vi "DAQ_E_mIO_DIO.reset.vi"(0 "i ref in":refnum<vi>, 3 "ms timeout (10000)":i32=10000, 5 "error in (no error)":errorcluster) -> (14 "i ref out":refnum<vi>, 17 "timed out":bool, 19 "error out":errorcluster)   [LabVIEW 2014, in "DAQ_E_mIO_DIO.lvlib"]
doc: "Sets all bits of the digital output port to 0.\n\nLicense Agreement for this software:\n\nCopyright (C)\nGesellschaft für Schwerionenforschung, GSI\nPlanckstr. 1\n64291 Darmstadt\nGermany\n\nContact: D.Beck@gsi.de \n\nThis program is free software; you can redistribute it and/or modify it under the terms of the GNU General Public License as published by the Free Software Foundation; either version 2 of the license, or (at your option) any later version.\n\nThis program is distributed in the hope that it will be useful, but WITHOUT ANY WARRANTY; without even the implied warranty of MERCHANTABILITY or FITNESS FOR A PARTICULAR PURPOSE. See the GNU General License for more details (http://www.gnu.org).\n\nGesellschaft für Schwerionenforschung, GSI\nPlanckstr. 1, 64291 Darmstadt, Germany\nFor all questions and ideas contact: M.Richter@gsi.de, H.Brand@gsi.de or D.Beck@gsi.de.\nLast update: 17-JUN-2004"
uses:
  DAQ_E_mIO_DIO.lvlib
  CS_Core/CSApplicationBaseClasses/DeviceBase/DeviceBase.lvlib
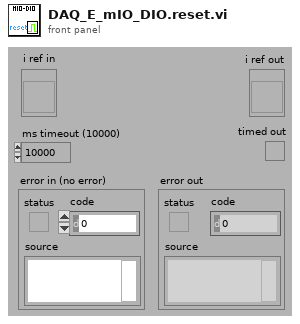
[diagram p1: front panel]
types:
  T1 = typedef "DAQ_E_mIO_DIO.lvlib/DAQ_E_mIO_DIO.i attribute.ctl" = cluster{"DOutChannel":refnum<k21>, "DInChannel":refnum<k21>, "nOfBitsIn":i32, "nOfBitsOut":i32}
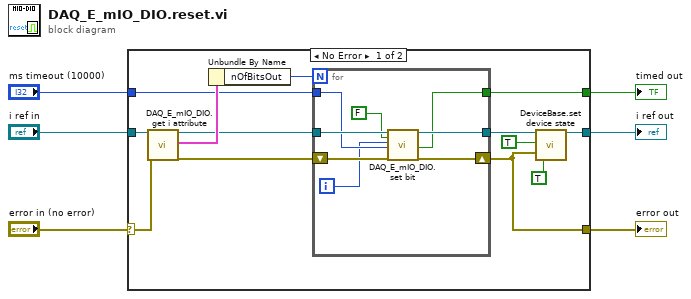
[diagram p0: block diagram]
diagram:
  n1 = case shown="No Error" "error in (no error)" {
    selector: "error in (no error)" -> [w17 w28]
    tunnel: "i ref in" -> [w19 w29]
    tunnel: "ms timeout (10000)" -> [w14 _]
    tunnel: [w13 _] -> w4
    tunnel: [w10 w29] -> w3
    tunnel: [w9 w28] -> w2
    frame No Error {
      n2 = call "DAQ_E_mIO_DIO.get i attribute.vi"("i ref in"=w19, "error in (no error)"=w17) -> ("i ref out"=w16:refnum<vi>, "i attribute"=w18:T1, "error out"=w15:errorcluster)  [unwired: 15 in]
      n3 = Unbundle By Name(w18) -> ("nOfBitsOut"=w12:i32)
      n4 = for {
        N: w12 -> [_]
        tunnel: w16 -> [w27]
        tunnel: w14 -> [w25]
        tunnel: [w22] -> w11
        tunnel: [w20] -> w13
        shift-right: [w21] -> w9
        shift-left: w15 -> [w26]
        i -> [w24]
        n5 = call "DAQ_E_mIO_DIO.set bit.vi"("i ref in"=w27, "bit"=FALSE, "bitNo"=w24, "ms timeout (10000)"=w25, "error in (no error)"=w26) -> ("i ref out"=w22:refnum<vi>, "timed out"=w20:bool, "error out"=w21:errorcluster)  [unwired: 12 in]
      }
      n6 = call "DeviceBase.set device state.vi"("i ref in"=w11, "implicit"=TRUE, "device error"=w9, "mayResetError (FALSE)"=TRUE) -> ("i ref out"=w10:refnum<vi>)  [unwired: 13 in, 2 out]
    }
    frame Error {
    }
  }
  "error out" <- w2
  "i ref out" <- w3
  "timed out" <- w4
